vi "TimingTest.vi"() -> ()   [LabVIEW 2011]
uses:
  BehaviorData/BehaviorData.lvclass
  Experiments/ClassDiscrimination/ClassDiscrimination.lvclass
  Electrophysiology/Electrophysiology.lvclass
  <vilib>/DAQmx/read.llb/DAQmx Read (Analog 2D DBL NChan NSamp).vi
  <vilib>/DAQmx/miscellaneous.llb/DAQmx Fill In Error Info.vi
panel:
  out "Ephys error":dbl
  out "Beh error":dbl
  out "Waveform Chart":dbl(graph)
  out "Sampling ratio":dbl
  in  "Recording Channels":refnum<k21>="State System Analog Input"
  out "error out 2":errorcluster
  out "error out":errorcluster
  out "Beh Samples per ms":dbl
  out "Ephys Samples per ms":dbl
  out "Counter Time":dbl
  out "Behavior Samples":i32
  in  "Recording Task":refnum<k21>="All4498"
  in  "Stop":bool
  out "Ephys Samples":dbl
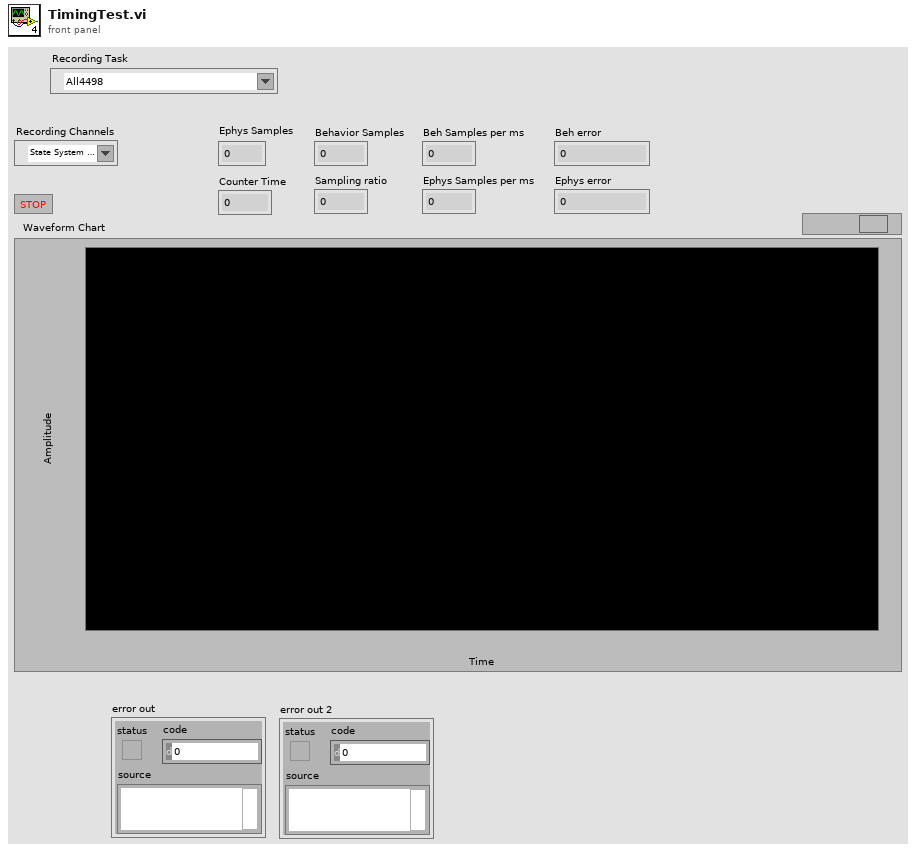
[diagram p1: front panel]
types:
  T1 = typedef "StimulationPrimary.ctl" = cluster{"setup":u8, "subject_id":i32, "session_start_time":dbl, "stim_start_time":dbl}
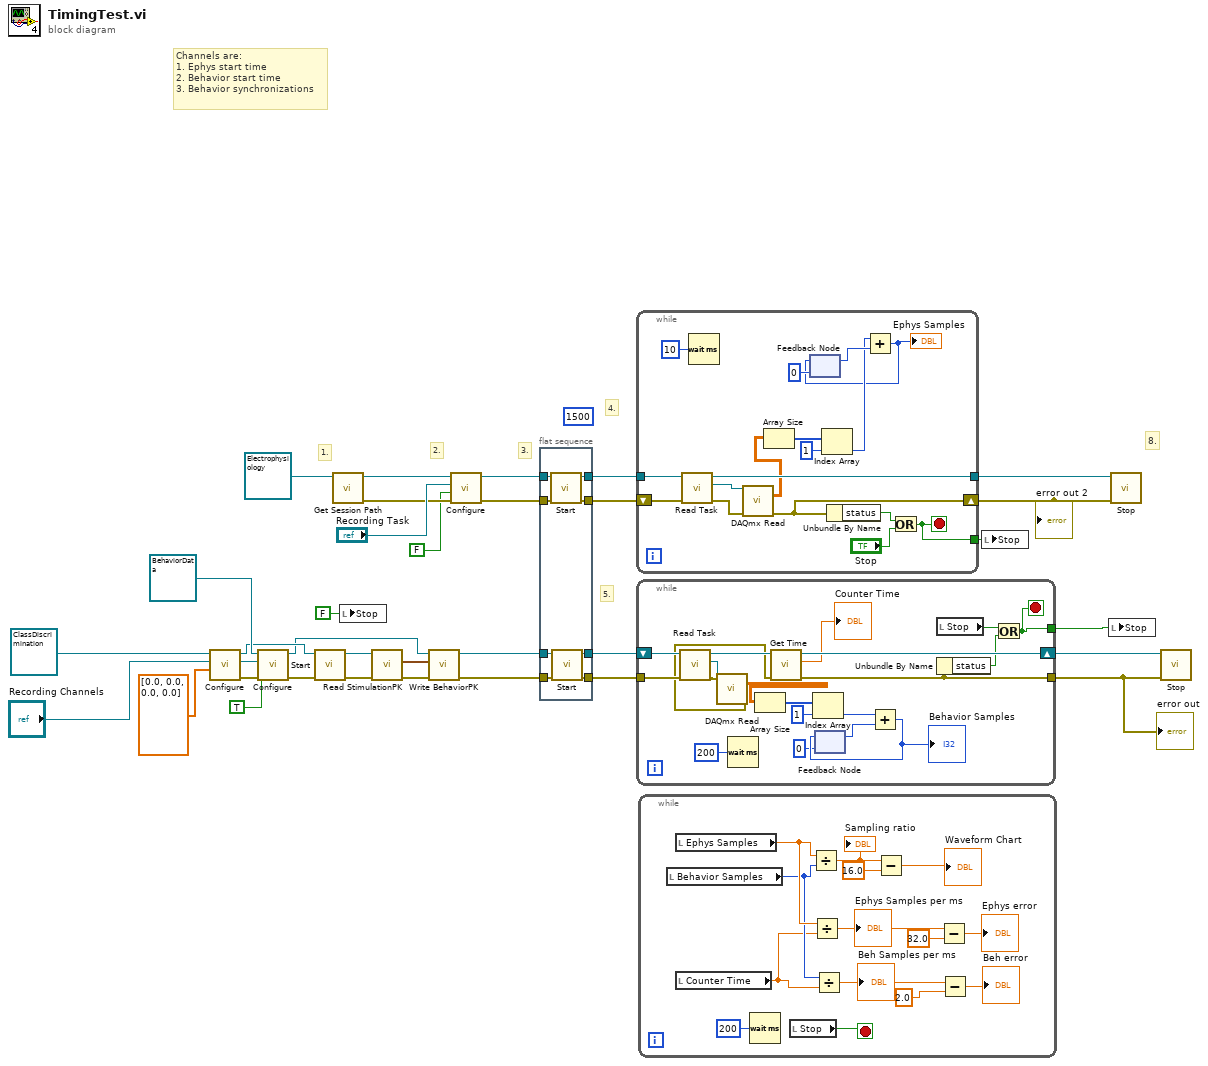
[diagram p0: block diagram]
diagram:
  (unwired) 1500 ("Read Size")
  # "5."
  # "8."
  # "3."
  # "2."
  # "1."
  # "4."
  # "Channels are:\n1. Ephys start time\n2. Behavior start time\n3. Behavior synchronizations"
  n1 = call-dynamic "Configure.vi"("Eye Params"=dbl[] [0.0, 0.0, 0.0, 0.0] ("Init Eye Params"), "TrialBasedExperiment in"=refnum<class "ClassDiscrimination.lvclass"> refnum ("ClassDiscrimination.lvclass")) -> ("error out"=w30:errorcluster, "TrialBasedExperiment out"=w29:refnum<class "ClassDiscrimination.lvclass">)  [unwired: 8 in]
  n2 = call-dynamic "Configure.vi"("error in (no error)"=w30, "Record"=TRUE, "Recording Channels"="Recording Channels", "BehaviorData in"=refnum<class "BehaviorData.lvclass"> refnum ("BehaviorData.lvclass")) -> ("error out"=w25:errorcluster, "BehaviorData out"=w23:refnum<class "BehaviorData.lvclass">)  [unwired: 6 in]
  n3 = call-dynamic "Start.vi"("error in (no error)"=w25, "TrialBasedExperiment in"=w29) -> ("error out"=w26:errorcluster, "TrialBasedExperiment out"=w27:refnum<class "ClassDiscrimination.lvclass">)  [unwired: 8 in]
  n4 = call-dynamic "Get Session Path.vi"("AcquistionObject in"=refnum<class "Electrophysiology.lvclass"> refnum ("Electrophysiology.lvclass")) -> ("error out"=w6:errorcluster, "AcquistionObject out"=w7:refnum<class "Electrophysiology.lvclass">)  [unwired: 8 in, 1 out]
  n5 = local write "Stop"(FALSE ("Stop")) -> ()
  n6 = call-dynamic "Read StimulationPK.vi"("error in (no error)"=w26, "TrialBasedExperiment in"=w27) -> ("error out"=w21:errorcluster, "StimulationPK"=w24:T1)  [unwired: 7 in, 1 out]
  n7 = call-dynamic "Write BehaviorPK.vi"("error in (no error)"=w21, "BehaviorPK"=w24, "BehaviorData in"=w23) -> ("error out"=w16:errorcluster, "BehaviorData out"=w22:refnum<class "BehaviorData.lvclass">)  [unwired: 7 in]
  n8 = call-dynamic "Configure.vi"("error in (no error)"=w6, "Record"=FALSE, "Recording Channels"="Recording Task", "Electrophysiology in"=w7) -> ("error out"=w2:errorcluster, "Electrophysiology out"=w3:refnum<class "Electrophysiology.lvclass">)  [unwired: 6 in]
  n9 = flat-sequence {
    tunnel: w22 -> [w41]
    tunnel: [w40] -> w20
    tunnel: [w39] -> w19
    tunnel: w16 -> [w38]
    tunnel: [w37] -> w12
    tunnel: [w36] -> w10
    tunnel: w3 -> [w35]
    tunnel: w2 -> [w34]
    frame #0 {
      n10 = call-dynamic "Start.vi"("error in (no error)"=w34, "Electrophysiology in"=w35) -> ("error out"=w36:errorcluster, "Electrophysiology out"=w37:refnum<class "Electrophysiology.lvclass">)  [unwired: 8 in]
      n11 = call-dynamic "Start.vi"("error in (no error)"=w38, "Electrophysiology in"=w41) -> ("error out"=w39:errorcluster, "Electrophysiology out"=w40:refnum<class "BehaviorData.lvclass">)  [unwired: 8 in]
    }
  }
  n12 = while {
    tunnel: w12 -> [w48]
    tunnel: [w46] -> w11
    tunnel: [w56] -> w4
    shift-right: [w43] -> w1
    shift-left: w10 -> [w47]
    stop <- w56 stop-if-true
    n13 = call-dynamic "Read Task.vi"("error in (no error)"=w47, "AcquireTraces in"=w48) -> ("error out"=w44:errorcluster, "Task"=w45:refnum<k21>, "AcquireTraces out"=w46:refnum<class "Electrophysiology.lvclass">)  [unwired: 7 in]
    n14 = Wait (ms)(milliseconds to wait=u32 10) -> ()  [unwired: 1 out]
    n15 = call-poly <vilib>:"DAQmx Read.vi"("task/channels in"=w45, "error in"=w44) -> ("data"=w42:dbl[][], "error out"=w43:errorcluster)  [unwired: 11 in, 1 out]
    n16 = Array Size(array=w42) -> (size(s)=w55:i32[])
    n17 = feedback #1(0) -> (w53:i32)
    n18 = Index Array(array=w55, index=1) -> (element=w51:i32)
    n19 = Unbundle By Name(w43) -> ("status"=w58:bool)
    n20 = Add(x=w51, y=w53) -> (x+y=w50:i32)
    "Ephys Samples" <- w50
    n21 = feedback-in #1(w50) -> ()
    n22 = Or(x=w58, y="Stop") -> (x .or. y?=w56:bool)
  }
  "error out 2" <- w1
  n23 = while {
    tunnel: [w70] -> w17
    tunnel: w19 -> [w64]
    shift-right: [w75] -> w18
    shift-left: w20 -> [w65]
    tunnel: [w67] -> w13
    stop <- w67 stop-if-true
    n24 = call-dynamic "Read Task.vi"("error in (no error)"=w64, "AcquireTraces in"=w65) -> ("error out"=w60:errorcluster, "Task"=w62:refnum<k21>, "AcquireTraces out"=w63:refnum<class "BehaviorData.lvclass">)  [unwired: 7 in]
    n25 = call-poly <vilib>:"DAQmx Read.vi"("task/channels in"=w62, "error in"=w60) -> ("data"=w61:dbl[][], "error out"=w59:errorcluster)  [unwired: 11 in, 1 out]
    n26 = Wait (ms)(milliseconds to wait=u32 200) -> ()  [unwired: 1 out]
    n27 = Array Size(array=w61) -> (size(s)=w73:i32[])
    n28 = call-dynamic "Get Time.vi"("error in (no error)"=w59, "BehaviorData in"=w63) -> ("error out"=w70:errorcluster, "Counter Time"=→"Counter Time":dbl, "BehaviorData out"=w75:refnum<class "BehaviorData.lvclass">)  [unwired: 7 in]
    n29 = Index Array(array=w73, index=1) -> (element=w71:i32)
    n30 = feedback #2(0) -> (w78:i32)
    n31 = Add(x=w71, y=w78) -> (x+y=w77:i32)
    "Behavior Samples" <- w77
    n32 = feedback-in #2(w77) -> ()
    n33 = local read "Stop"() -> (w69:bool)
    n34 = Unbundle By Name(w70) -> ("status"=w68:bool)
    n35 = Or(x=w69, y=w68) -> (x .or. y?=w67:bool)
  }
  "error out" <- w17
  n36 = while {
    stop <- w92 stop-if-true
    n37 = local read "Behavior Samples"() -> (w87:i32)
    n38 = local read "Ephys Samples"() -> (w88:dbl)
    n39 = local read "Counter Time"() -> (w86:dbl)
    n40 = Wait (ms)(milliseconds to wait=u32 200) -> ()  [unwired: 1 out]
    n41 = local read "Stop"() -> (w92:bool)
    n42 = Divide(x=w88, y=w87) -> (x/y=w91:dbl)
    "Sampling ratio" <- w91
    n43 = Divide(x=w88, y=w86) -> (x/y=w81:dbl)
    "Ephys Samples per ms" <- w81
    n44 = Divide(x=w87, y=w86) -> (x/y=w84:dbl)
    "Beh Samples per ms" <- w84
    n45 = Subtract(x=w91, y=16.0) -> (x-y=→"Waveform Chart":dbl)
    n46 = Subtract(x=w81, y=32.0) -> (x-y=→"Ephys error":dbl)
    n47 = Subtract(x=w84, y=2.0) -> (x-y=→"Beh error":dbl)
  }
  n48 = local write "Stop"(w4) -> ()
  n49 = local write "Stop"(w13) -> ()
  n50 = call-dynamic "Stop.vi"("error in (no error)"=w1, "Electrophysiology in"=w11) -> ()  [unwired: 8 in, 2 out]
  n51 = call-dynamic "Stop.vi"("error in (no error)"=w17, "Electrophysiology in"=w18) -> ()  [unwired: 8 in, 2 out]
